vi "Format IBE.vi"(10 "IBEMissionsion":T1={"MeasurementStatus"=enum."FAIL", "ReferenceChannelPower"=0.0, "UpperChannelTotalPower"=0.0, "LowerChannelTotalPower"=0.0, "TotalChannelPower"=[]}) -> (2 "IBE Results":T2)   [LabVIEW 2015, in "niDTS BT.lvlib" / "niDTS BT INSTR TX.lvclass"]
uses:
  niDTS BT INSTR TX.lvclass
  Tests/Tx Test/Includes/niDTS BT Tx Test INC IBE Results.ctl
  niDTS BT.lvlib
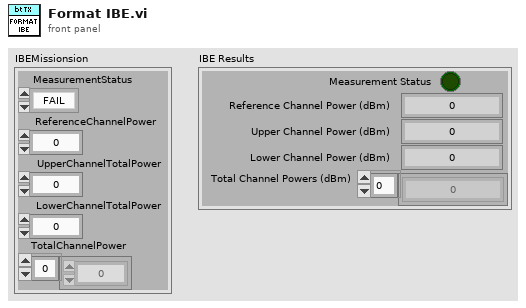
[diagram p1: front panel]
types:
  T1 = cluster{"MeasurementStatus":enum16{"PASS", "FAIL"}, "ReferenceChannelPower":dbl, "UpperChannelTotalPower":dbl, "LowerChannelTotalPower":dbl, "TotalChannelPower":dbl[]}
  T2 = typedef "niDTS BT.lvlib/niDTS BT Tx Test INC IBE Results.ctl" = cluster{"Measurement Status":bool, "Reference Channel Power (dBm)":dbl, "Upper Channel Power (dBm)":dbl, "Lower Channel Power (dBm)":dbl, "Total Channel Powers (dBm)":dbl[]}
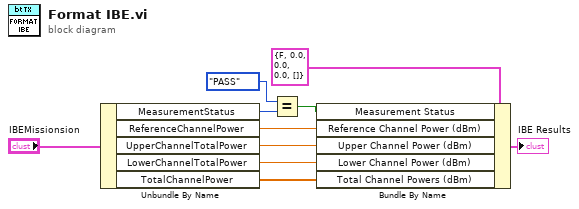
[diagram p0: block diagram]
diagram:
  n1 = Unbundle By Name("IBEMissionsion") -> ("MeasurementStatus"=w6:enum16{"PASS", "FAIL"}, "ReferenceChannelPower"=w2:dbl, "UpperChannelTotalPower"=w3:dbl, "LowerChannelTotalPower"=w4:dbl, "TotalChannelPower"=w5:dbl[])
  n2 = Equal?(x=enum16{"PASS", "FAIL"}."PASS", y=w6) -> (x = y?=w8:bool)
  n3 = Bundle By Name(cluster=T2 {"Measurement Status"=FALSE, "Reference Channel Power (dBm)"=0.0, "Upper Channel Power (dBm)"=0.0, "Lower Channel Power (dBm)"=0.0, "Total Channel Powers (dBm)"=[]} ("IBE Results"), "Measurement Status"=w8, "Reference Channel Power (dBm)"=w2, "Upper Channel Power (dBm)"=w3, "Lower Channel Power (dBm)"=w4, "Total Channel Powers (dBm)"=w5) -> (→"IBE Results":T2)
